vi "Obtain Tif files in folder.vi"(8 "error in":errorcluster, 11 "Z-stack images folder path":path) -> (0 "error IO":errorcluster, 2 "Tif files paths":path[](array[path]), 3 "filenames (no extension)":string[](array[string]))   [LabVIEW 2013]
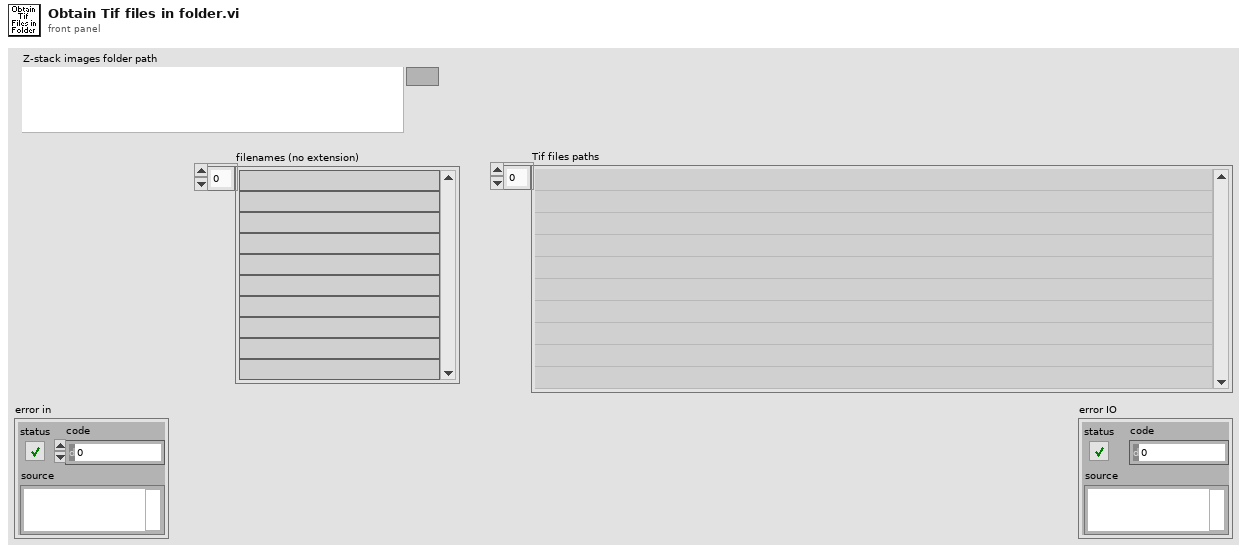
[diagram p1: front panel]
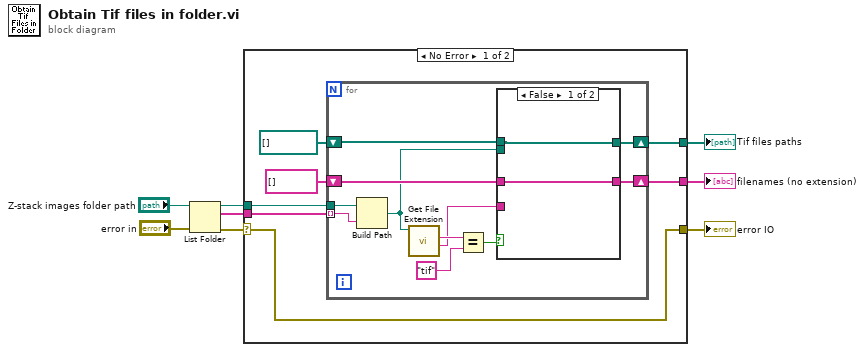
[diagram p0: block diagram]
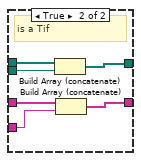
[diagram p2: hidden frame]
diagram:
  n1 = List Folder(path="Z-stack images folder path", error in="error in") -> (path out=w7:path, filenames=w6:string[], error out=w3:errorcluster)  [unwired: 2 in, 1 out]
  n2 = case shown="No Error" w3 {
    selector: w3 -> [w11 w35]
    tunnel: [w15 _] -> w8
    tunnel: w7 -> [w13 _]
    tunnel: w6 -> [w12 _]
    tunnel: [w11 w35] -> w2
    tunnel: [w9 _] -> w1
    frame No Error {
      n3 = for {
        tunnel: w12 -> [w26] mode=indexing
        tunnel: w13 -> [w25]
        shift-right: [w21] -> w15
        shift-left: string[] [] -> [w20]
        shift-right: [w17] -> w9
        shift-left: path[] [] -> [w16]
        n4 = Build Path(base path=w25, name or relative path=w26) -> (appended path=w18:path)
        n5 = call <vilib>:"Get File Extension.vi"("file"=w18) -> ("filename without extension"=w19:string, "lowercase file extension"=w22:string)  [unwired: 7 in, 2 out]
        n6 = Equal?(x=w22, y="tif") -> (x = y?=w23:bool)
        n7 = case shown="False" w23 {
          tunnel: [w28 w34] -> w21
          tunnel: w20 -> [w28 w33]
          tunnel: w19 -> [_ w32]
          tunnel: w18 -> [_ w31]
          tunnel: [w27 w30] -> w17
          tunnel: w16 -> [w27 w29]
          frame False {
          }
          frame True {
            # "is a Tif"
            n8 = Build Array (concatenate)(w29, w31) -> (w30:path[])
            n9 = Build Array (concatenate)(w33, w32) -> (w34:string[])
          }
        }
      }
    }
    frame Error {
    }
  }
  "filenames (no extension)" <- w8
  "error IO" <- w2
  "Tif files paths" <- w1
